vi "IsHotGoalDB.vi"(7 "Timeout (ms)":u32, 8 "error in":errorcluster, 9 "DBHot?":string="Boolean", 10 "DBFinished?":string="Boolean", 11 "DBStart":string="Boolean") -> (0 "error out":errorcluster, 1 "TimedOut?":bool, 2 "Hot?":bool)   [LabVIEW 2013]
doc: "IsHotGoalDB determines whether or not the goal is hot. Image processing is done on the laptop (through the DB).\n-DBStart: the name of the DB boolean control that starts image processing. IsHotGoalDB writes to this to signal the DB to start.\n-DBFinished?: the name of the DB boolean indicator that indicates when the DB is done processing.\n-DBHot?: the name of the DB boolean indicator that indicates whether the goal is hot."
panel:
  in  "milliseconds to wait":u32=20
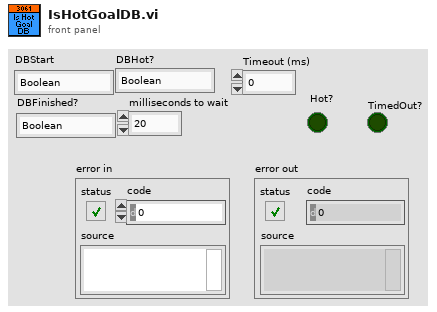
[diagram p1: front panel]
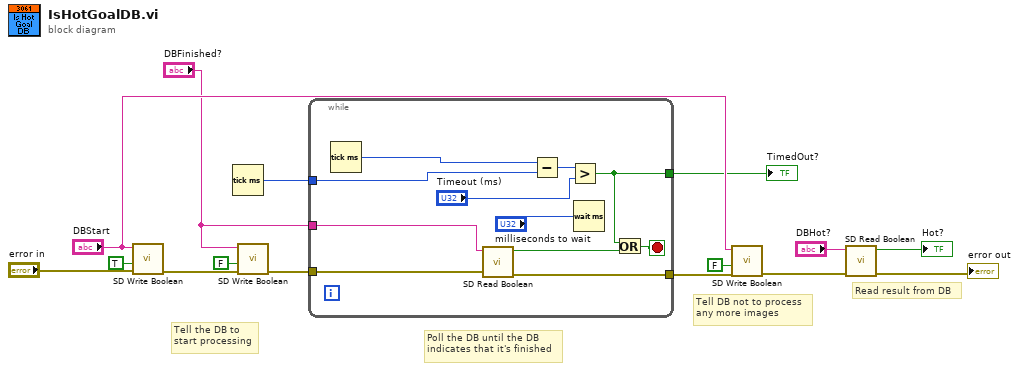
[diagram p0: block diagram]
diagram:
  # "Tell DB not to process\nany more images"
  # "Read result from DB"
  # "Poll the DB until the DB\nindicates that it's finished"
  # "Tell the DB to\nstart processing"
  n1 = call <vilib>:"SD Write Boolean.vi"("error in"="error in", "Boolean"=TRUE, "Name"="DBStart") -> ("error out"=w6:errorcluster)  [unwired: 7 in, 1 out]
  n2 = Tick Count (ms)() -> (millisecond timer value=w2:u32)
  n3 = call <vilib>:"SD Write Boolean.vi"("error in"=w6, "Boolean"=FALSE, "Name"="DBFinished?") -> ("error out"=w5:errorcluster)  [unwired: 7 in, 1 out]
  n4 = while {
    tunnel: w5 -> [w26]
    tunnel: [w25] -> w9
    tunnel: "DBFinished?" -> [w24]
    tunnel: w2 -> [w19]
    tunnel: [w16] -> w1
    stop <- w22 stop-if-true
    n5 = Tick Count (ms)() -> (millisecond timer value=w20:u32)
    n6 = call <vilib>:"SD Read Boolean.vi"("error in"=w26, "Name"=w24) -> ("error out"=w25:errorcluster, "Boolean"=w21:bool)  [unwired: 7 in, 1 out]
    n7 = Subtract(x=w20, y=w19) -> (x-y=w18:u32)
    n8 = Greater?(x=w18, y="Timeout (ms)") -> (0:w16:bool)
    n9 = Wait (ms)(milliseconds to wait="milliseconds to wait") -> ()  [unwired: 1 out]
    n10 = Or(x=w16, y=w21) -> (x .or. y?=w22:bool)
  }
  "TimedOut?" <- w1
  n11 = call <vilib>:"SD Write Boolean.vi"("error in"=w9, "Boolean"=FALSE, "Name"="DBStart") -> ("error out"=w8:errorcluster)  [unwired: 7 in, 1 out]
  n12 = call <vilib>:"SD Read Boolean.vi"("error in"=w8, "Name"="DBHot?") -> ("error out"=→"error out":errorcluster, "Boolean"=→"Hot?":bool)  [unwired: 7 in, 1 out]
